vi "Reset MotorSim.vi"(8 "error in (no error)":errorcluster, 11 "Motor in":refnum<class "Motor.lvclass">) -> (0 "error out":errorcluster, 3 "Motor out":refnum<class "Motor.lvclass">)   [LabVIEW 2018, in "Motor.lvclass"]
uses:
  Motor.lvclass
  Motor.lvclass/Motor.ctl
  StateManager/StateManager.lvclass/StateManager.ctl
  MotorSim/MotorSim.lvclass
  StateManager/StateManager.lvclass
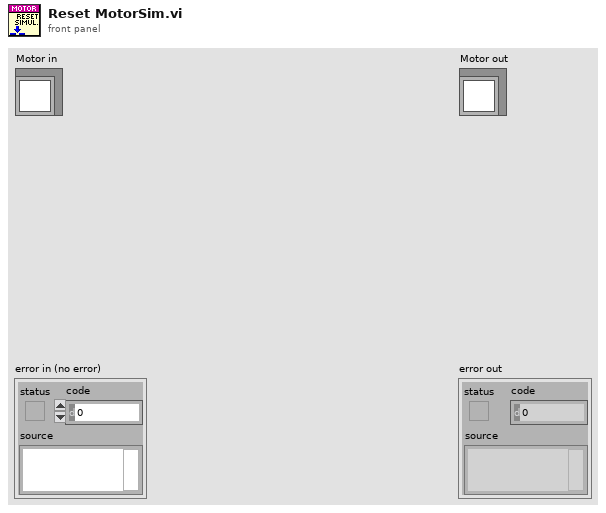
[diagram p1: front panel]
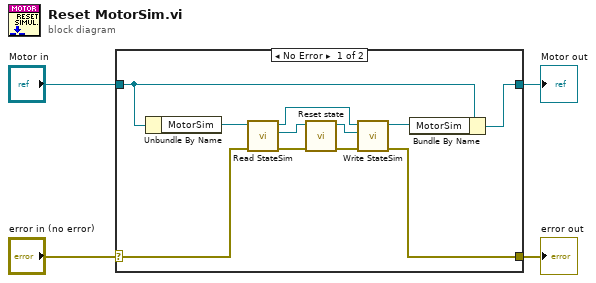
[diagram p0: block diagram]
diagram:
  n1 = case shown="No Error" "error in (no error)" {
    selector: "error in (no error)" -> [w14 w16]
    tunnel: [w5 w16] -> w3
    tunnel: [w6 w17] -> w1
    tunnel: "Motor in" -> [w8 w17]
    frame No Error {
      n2 = Unbundle By Name(w8) -> ("MotorSim"=w15:refnum<class "MotorSim.lvclass">)
      n3 = call-dynamic "Read StateSim.vi"("error in (no error)"=w14, "MotorSim in"=w15) -> ("error out"=w13:errorcluster, "StateSim"=w12:refnum<class "StateManager.lvclass">, "MotorSim out"=w9:refnum<class "MotorSim.lvclass">)  [unwired: 6 in, 1 out]
      n4 = call "Reset state.vi"("error in (no error)"=w13, "StateManager in"=w12) -> ("error out"=w11:errorcluster, "StateManager out"=w10:refnum<class "StateManager.lvclass">)  [unwired: 8 in]
      n5 = call-dynamic "Write StateSim.vi"("error in (no error)"=w11, "StateSim"=w10, "MotorSim in"=w9) -> ("error out"=w5:errorcluster, "MotorSim out"=w7:refnum<class "MotorSim.lvclass">)  [unwired: 7 in]
      n6 = Bundle By Name(cluster=w8, "MotorSim"=w7) -> (w6:refnum<class "Motor.lvclass">)
    }
    frame Error {
    }
  }
  "error out" <- w3
  "Motor out" <- w1
